vi "config fpga resource.vi"(0 "fifo channel in":refnum<class "fifo channel.lvclass">, 1 "pairs in":T2[](array[typedef]), 2 "tagbus index":i32, 3 "bitfile ref in":refnum<k20>, 4 "hardware resource":T1, 5 "error in (no error)":errorcluster) -> (14 "fifo channel out":refnum<class "fifo channel.lvclass">, 15 "pairs out":T2[](array[typedef]), 19 "error out":errorcluster)   [LabVIEW 2014, in "fifo channel.lvclass"]
uses:
  fifo channel.lvclass
  OLD Project Folder/execution/control index set.ctl
  <vilib>/NI/Tag Bus/tag/Data Type.ctl
  OLD Project Folder/configuration/fpga resource supported data types.ctl
  <vilib>/NI/LVFPGA Adv Session Resources/ResourceInfo.ctl
  <vilib>/NI/Tag Bus/tag/tag descriptor.lvclass/tag descriptor.ctl
  fifo channel.lvclass/fifo channel.ctl
  <vilib>/NI/LVFPGA Adv Session Resources/OpenByNameSubVI.vi
  <vilib>/NI/Tag Bus/tag/read data type.vi
  <vilib>/NI/Tag Bus/tag/read tag name.vi
  Read fifo config.vi
  <vilib>/rvi/interface/common/dynamic/niFpgaEscapeDelimiterAndNull.vi
  <vilib>/Utility/error.llb/Error Cluster From Error Code.vi
  <vilib>/rvi/interface/common/niFpgaWaitOnOcc.vi
  <vilib>/NI/LVFPGA Adv Session Resources/OpenByName.xnode
  <vilib>/rvi/interface/nirviMethod/nirviMethod.xnode
  <vilib>/rvi/errors/niLvFpgaMergeErrorWithErrorCode.vi
  OLD Project Folder/execution/io runtime.lvclass
  fpga channel/fpga channel.lvclass
  <vilib>/NI/Tag Bus/tag/tag descriptor.lvclass
  <vilib>/FPGAPlugInAG/Dynamic/niLvFpga_ConfigureFifo_Dynamic.vi
  <vilib>/FPGAPlugInAG/Dynamic/niLvFpga_StartFifo_Dynamic.vi
  <vilib>/NI/LVFPGA Adv Session Resources/LVFPGAAdvSessionResources.lvlib
  <vilib>/Utility/VariantDataType/VariantType.lvlib
panel:
  out "Actual Depth":u32
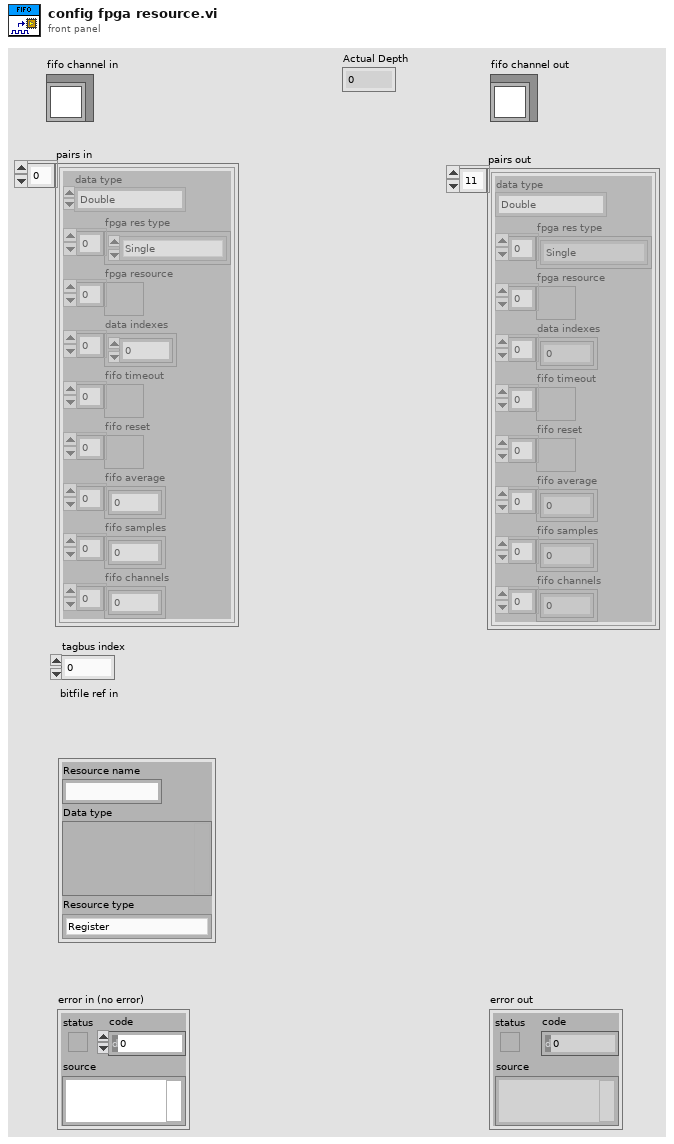
[diagram p1: front panel]
types:
  T1 = typedef "LVFPGAAdvSessionResources.lvlib/ResourceInfo.ctl" = cluster{"Resource name":string, "Data type":variant, "Resource type":enum16{"Register", "Host To Target FIFO", "Target To Host FIFO"}}
  T2 = typedef "io runtime.lvclass/control index set.ctl" = cluster{"data type":T3, "fpga res type":T4[], "fpga resource":refnum<k20>[], "data indexes":i32[], "fifo timeout":refnum<k20>[], "fifo reset":refnum<k20>[], "fifo average":i32[], "fifo samples":u32[], "fifo channels":u32[]}
  T3 = typedef "tag bus.lvlib/tag descriptor.lvclass/Data Type.ctl" = enum16{"Double", "Single", "I64", "I32", "I16", "I8", "U64", "U32", "U16", "U8", "Boolean", "String", "Array of Double", "Array of Single", "Array of I64", "Array of I32", "Array of I16", "Array of I8", "Array of U64", "Array of U32", "Array of U16", "Array of U8", "Array of Boolean", "Array of String"}
  T4 = typedef "fpga channel.lvclass/fpga resource supported data types.ctl" = enum16{"Invalid Type", "Single", "I64", "I32", "I16", "I8", "U64", "U32", "U16", "U8", "Boolean", "FXP I,20,5", "FXP I,24,5", "FXP I,24,10", "Fifo 1023,I16"}
  T5 = typedef "fifo channel.lvclass/fifo channel settings.ctl" = cluster{"Timeout":string, "Reset":string, "Averages":i32, "Samples":u32, "Channels":i32, "Fifo size":u32}
  T6 = cluster{"Name":string, "Depth":u32, "Write? (Deprecated:Use Implementation)":bool, "Physical Channel":u32, "Base Address":u32, "Data Width":u32, "Data Type":enum32{"Boolean", "I8", "I16", "I32", "I64", "U8", "U16", "U32", "U64", "FXP", "CustomControl", "SGL"}, "FXP Properties":variant, "Write Window Address":u32, "Implementation":enum16{"niFpgaTargetToHost", "niFpgaHostToTarget", "niFpgaPeerToPeerWriter", "niFpgaPeerToPeerReader", "niCoreTargetToHost", "niCoreHostToTarget"}, "Control Set":u32}[]
  T7 = cluster{"Name":string, "type":variant, "indicator?":bool}[]
  T8 = typedef "VariantType.lvlib/Type.ctl" = enum8{"Invalid Type", "Void", "I8", "I16", "I32", "I64", "U8", "U16", "U32", "U64", "Single Float", "Double Float", "Extended Float", "Single Complex", "Double Complex", "Extended Complex", "Enum U8", "Enum U16", "Enum U32", "Enum U64", "Single Float With Unit", "Double Float With Unit", "Extended Float With Unit", "Single Complex with Unit", "Double Complex with Unit", "Extended Complex with Unit", "Boolean", "String", "Path", "Picture", "Tag", "Array", "Cluster", "Variant", "LV Variant", "Waveform", "Timestamp", "Digital Waveform", "Digital Data", "ExpressData", "Refnum", "External Data", "VI", "Poly VI", "LabVIEW Class Instance", "Fixed Point"}
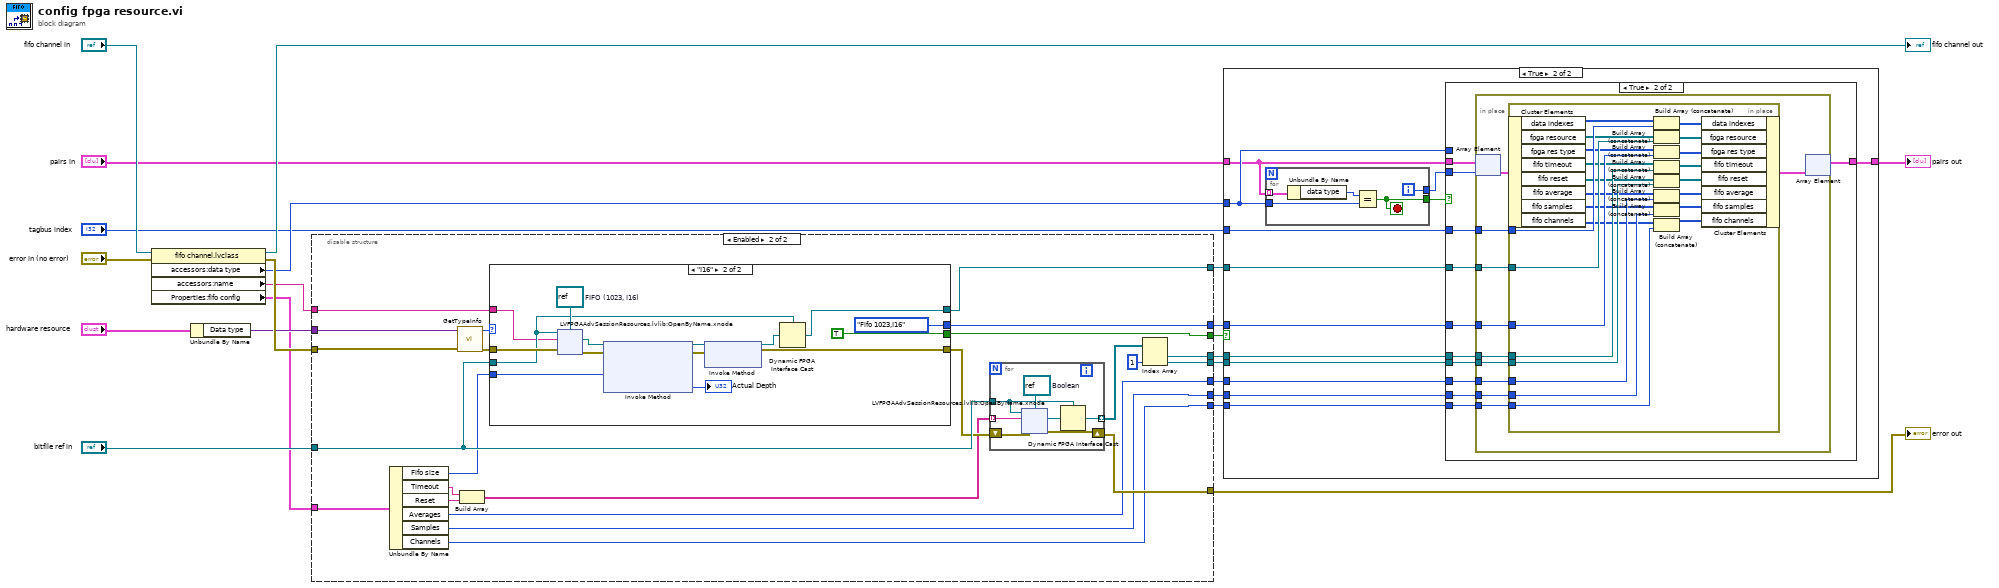
[diagram p0: block diagram]
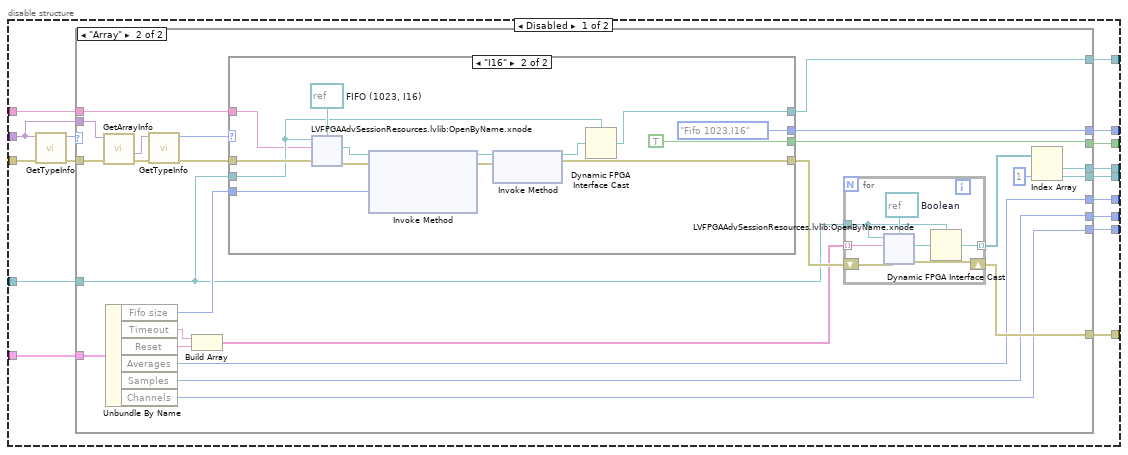
[diagram p2: hidden frame]
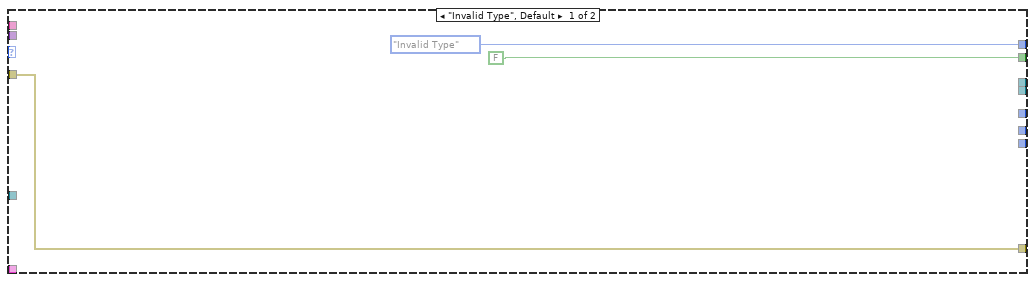
[diagram p3: hidden frame]
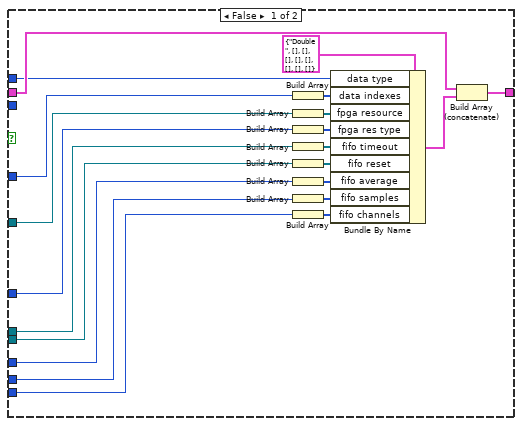
[diagram p7: hidden frame]
diagram:
  n1 = property class="fifo channel.lvclass"(reference="fifo channel in", error in="error in (no error)") -> (reference out=→"fifo channel out":refnum<class "fifo channel.lvclass">, error out=w22:errorcluster, "accessors:data type"=w19:T3, "accessors:name"=w10:string, "Properties:fifo config"=w11:T5)
  n2 = Unbundle By Name("hardware resource") -> ("Data type"=w14:variant)
  n3 = disable-structure shown="Enabled" {
    disable-tunnel: w22 -> [w38 w116]
    disable-tunnel: w14 -> [w36 w117]
    disable-tunnel: "bitfile ref in" -> [w35 w138]
    disable-tunnel: w11 -> [w34 w137]
    disable-tunnel: w10 -> [w33 w136]
    disable-tunnel: [w32 w135] -> w9
    disable-tunnel: [w31 w134] -> w8
    disable-tunnel: [w30 w133] -> w7
    disable-tunnel: [w29 w132] -> w6
    disable-tunnel: [w28 w131] -> w5
    disable-tunnel: [w27 w130] -> w4
    disable-tunnel: [w26 w129] -> w3
    disable-tunnel: [w25 w128] -> w2
    disable-tunnel: [w24 w127] -> w1
    frame Disabled {
      n4 = call <vilib>:"GetTypeInfo.vi"("error in (no error)"=w38, "Variant"=w36) -> ("error out"=w37:errorcluster, "Type Enum"=w23:T8)  [unwired: 5 in, 3 out]
      n5 = case shown="\"Array\"" w23 {
        tunnel: w37 -> [w39 w62]
        tunnel: [FALSE w50] -> w32
        tunnel: w36 -> [_ w61]
        tunnel: w35 -> [_ w53]
        tunnel: [fpga_resource_supported_data_types."Invalid Type" ("fpga res type") w51] -> w29
        tunnel: w34 -> [_ w58]
        tunnel: w33 -> [_ w56]
        tunnel: [_ w52] -> w30
        tunnel: [w39 w49] -> w31
        tunnel: [_ w46] -> w28
        tunnel: [_ w45] -> w27
        tunnel: [_ w44] -> w26
        tunnel: [_ w43] -> w25
        tunnel: [_ w42] -> w24
        frame "Invalid Type", Default {
        }
        frame "Array" {
          n6 = call <vilib>:"GetArrayInfo.vi"("error in (no error)"=w62, "Variant"=w61) -> ("error out"=w64:errorcluster, "ArrayElement"=w63:variant)  [unwired: 6 in, 2 out]
          n7 = Unbundle By Name(w58) -> ("Fifo size"=w57:u32, "Timeout"=w55:string, "Reset"=w54:string, "Averages"=w44:i32, "Samples"=w43:u32, "Channels"=w42:i32)
          n8 = call <vilib>:"GetTypeInfo.vi"("error in (no error)"=w64, "Variant"=w63) -> ("error out"=w60:errorcluster, "Type Enum"=w65:T8)  [unwired: 5 in, 3 out]
          n9 = Build Array(w55, w54) -> (w59:string[])
          n10 = case shown="\"I16\"" w65 {
            tunnel: [_ TRUE] -> w50
            tunnel: w53 -> [_ w93]
            tunnel: w60 -> [w87 w94]
            tunnel: [w87 w92] -> w66
            tunnel: [_ fpga_resource_supported_data_types."Fifo 1023,I16" ("fpga res type")] -> w51
            tunnel: w57 -> [_ w91]
            tunnel: w56 -> [_ w90]
            tunnel: [_ w88] -> w52
            frame "Invalid Type", Default {
            }
            frame "I16" {
              w97 = refnum<k20> refnum  # FIFO (1023, I16)
              n11 = xnode "LVFPGAAdvSessionResources.lvlib:OpenByName.xnode"("FPGA VI Reference in"=w93, "Resource name in"=w90, "Single resource reference type in"=w97, "Error in"=w94) -> ("Single resource reference out"=w95:refnum<k20>, "Error out"=w100:errorcluster)  [unwired: 1 out]
              n12 = xnode "Invoke Method"("FPGA VI Reference In"=w95, "error in"=w100, "Requested Depth"=w91) -> ("FPGA VI Reference Out"=w98:refnum<k20>, "error out"=w99:errorcluster, "Actual Depth"=w89:u32)
              n13 = xnode "Invoke Method"("FPGA VI Reference In"=w98, "error in"=w99) -> ("FPGA VI Reference Out"=w96:refnum<k20>, "error out"=w92:errorcluster)
              n14 = Dynamic FPGA Interface Cast(Session In=w93, Type=w96) -> (Session Out=w88:refnum<k20>)
            }
          }
          n15 = for {
            shift-right: [w70] -> w49
            shift-left: w66 -> [w71]
            tunnel: w59 -> [w69] mode=indexing
            tunnel: [w68] -> w47 mode=indexing
            tunnel: w53 -> [w67]
            w73 = refnum<k20> refnum  # Boolean
            n16 = xnode "LVFPGAAdvSessionResources.lvlib:OpenByName.xnode"("FPGA VI Reference in"=w67, "Resource name in"=w69, "Single resource reference type in"=w73, "Error in"=w71) -> ("Single resource reference out"=w72:refnum<k20>, "Error out"=w70:errorcluster)  [unwired: 1 out]
            n17 = Dynamic FPGA Interface Cast(Session In=w67, Type=w72) -> (Session Out=w68:refnum<k20>)
          }
          n18 = Index Array(array=w47, index #2=1 ("index")) -> (element #1=w46:refnum<k20>, element #2=w45:refnum<k20>)  [unwired: 1 in]
        }
      }
    }
    frame Enabled {
      n19 = Unbundle By Name(w137) -> ("Fifo size"=w122:u32, "Timeout"=w121:string, "Reset"=w120:string, "Averages"=w129:i32, "Samples"=w128:u32, "Channels"=w127:i32)
      n20 = call <vilib>:"GetTypeInfo.vi"("error in (no error)"=w116, "Variant"=w117) -> ("error out"=w124:errorcluster, "Type Enum"=w125:T8)  [unwired: 5 in, 3 out]
      n21 = Build Array(w121, w120) -> (w123:string[])
      n22 = case shown="\"I16\"" w125 {
        tunnel: [_ TRUE] -> w135
        tunnel: w138 -> [_ w165]
        tunnel: w124 -> [w159 w166]
        tunnel: [w159 w164] -> w126
        tunnel: [_ fpga_resource_supported_data_types."Fifo 1023,I16" ("fpga res type")] -> w132
        tunnel: w122 -> [_ w163]
        tunnel: w136 -> [_ w162]
        tunnel: [_ w161] -> w133
        frame "Invalid Type", Default {
        }
        frame "I16" {
          w169 = refnum<k20> refnum  # FIFO (1023, I16)
          n23 = xnode "LVFPGAAdvSessionResources.lvlib:OpenByName.xnode"("FPGA VI Reference in"=w165, "Resource name in"=w162, "Single resource reference type in"=w169, "Error in"=w166) -> ("Single resource reference out"=w167:refnum<k20>, "Error out"=w172:errorcluster)  [unwired: 1 out]
          n24 = xnode "Invoke Method"("FPGA VI Reference In"=w167, "error in"=w172, "Requested Depth"=w163) -> ("FPGA VI Reference Out"=w170:refnum<k20>, "error out"=w171:errorcluster, "Actual Depth"=→"Actual Depth":u32)
          n25 = xnode "Invoke Method"("FPGA VI Reference In"=w170, "error in"=w171) -> ("FPGA VI Reference Out"=w168:refnum<k20>, "error out"=w164:errorcluster)
          n26 = Dynamic FPGA Interface Cast(Session In=w165, Type=w168) -> (Session Out=w161:refnum<k20>)
        }
      }
      n27 = for {
        shift-right: [w142] -> w134
        shift-left: w126 -> [w143]
        tunnel: w123 -> [w141] mode=indexing
        tunnel: [w140] -> w118 mode=indexing
        tunnel: w138 -> [w139]
        w145 = refnum<k20> refnum  # Boolean
        n28 = xnode "LVFPGAAdvSessionResources.lvlib:OpenByName.xnode"("FPGA VI Reference in"=w139, "Resource name in"=w141, "Single resource reference type in"=w145, "Error in"=w143) -> ("Single resource reference out"=w144:refnum<k20>, "Error out"=w142:errorcluster)  [unwired: 1 out]
        n29 = Dynamic FPGA Interface Cast(Session In=w139, Type=w144) -> (Session Out=w140:refnum<k20>)
      }
      n30 = Index Array(array=w118, index #2=1 ("index")) -> (element #1=w131:refnum<k20>, element #2=w130:refnum<k20>)  [unwired: 1 in]
    }
  }
  "error out" <- w8
  n31 = case shown="True" w9 {
    tunnel: [w188 w199] -> w20
    tunnel: w19 -> [_ w198]
    tunnel: "pairs in" -> [w188 w197]
    tunnel: "tagbus index" -> [_ w196]
    tunnel: w7 -> [_ w195]
    tunnel: w6 -> [_ w194]
    tunnel: w5 -> [_ w193]
    tunnel: w4 -> [_ w192]
    tunnel: w3 -> [_ w191]
    tunnel: w2 -> [_ w190]
    tunnel: w1 -> [_ w189]
    frame False {
    }
    frame True {
      n32 = for {
        tunnel: w197 -> [w272] mode=indexing
        tunnel: w198 -> [w270]
        tunnel: [w269] -> w201
        tunnel: [w268] -> w200
        i -> [w269]
        stop <- w268 stop-if-true
        n33 = Unbundle By Name(w272) -> ("data type"=w271:T3)
        n34 = Equal?(x=w271, y=w270) -> (x = y?=w268:bool)
      }
      n35 = case shown="True" w200 {
        tunnel: w197 -> [w222 w233]
        tunnel: [w221 w232] -> w199
        tunnel: w201 -> [_ w231]
        tunnel: w198 -> [w220 _]
        tunnel: w196 -> [w217 w230]
        tunnel: w195 -> [w215 w229]
        tunnel: w194 -> [w213 w228]
        tunnel: w193 -> [w211 w227]
        tunnel: w192 -> [w209 w226]
        tunnel: w191 -> [w207 w225]
        tunnel: w190 -> [w205 w224]
        tunnel: w189 -> [w203 w223]
        frame False {
          n36 = Build Array(w217) -> (w216:i32[])
          n37 = Build Array(w215) -> (w214:refnum<k20>[])
          n38 = Build Array(w213) -> (w212:T4[])
          n39 = Build Array(w211) -> (w210:refnum<k20>[])
          n40 = Build Array(w209) -> (w208:refnum<k20>[])
          n41 = Build Array(w207) -> (w206:i32[])
          n42 = Build Array(w205) -> (w204:u32[])
          n43 = Build Array(w203) -> (w202:i32[])
          n44 = Bundle By Name(cluster=T2 {"data type"=enum."Double", "fpga res type"=[], "fpga resource"=[], "data indexes"=[], "fifo timeout"=[], "fifo reset"=[], "fifo average"=[], "fifo samples"=[], "fifo channels"=[]} ("control index set"), "data type"=w220, "data indexes"=w216, "fpga resource"=w214, "fpga res type"=w212, "fifo timeout"=w210, "fifo reset"=w208, "fifo average"=w206, "fifo samples"=w204, "fifo channels"=w202) -> (w218:T2)
          n45 = Build Array (concatenate)(w222, w218) -> (w221:T2[])
        }
        frame True {
          n46 = in-place {
            in-place-border: w230 -> [w241]
            in-place-border: w229 -> [w240]
            in-place-border: w228 -> [w239]
            in-place-border: w227 -> [w238]
            in-place-border: w226 -> [w237]
            in-place-border: w225 -> [w236]
            in-place-border: w224 -> [w235]
            in-place-border: w223 -> [w234]
            n47 = in-place-array #1(w233, w231) -> (w243:T2)
            n48 = in-place {
              in-place-border: w241 -> [w265]
              in-place-border: w240 -> [w263]
              in-place-border: w239 -> [w260]
              in-place-border: w238 -> [w258]
              in-place-border: w237 -> [w254]
              in-place-border: w236 -> [w251]
              in-place-border: w235 -> [w247]
              in-place-border: w234 -> [w245]
              n49 = in-place-cluster #2(w243) -> ("data indexes"=w267:i32[], "fpga resource"=w264:refnum<k20>[], "fpga res type"=w261:T4[], "fifo timeout"=w257:refnum<k20>[], "fifo reset"=w255:refnum<k20>[], "fifo average"=w252:i32[], "fifo samples"=w249:u32[], "fifo channels"=w246:u32[])
              n50 = Build Array (concatenate)(w267, w265) -> (w266:i32[])
              n51 = Build Array (concatenate)(w264, w263) -> (w262:refnum<k20>[])
              n52 = Build Array (concatenate)(w261, w260) -> (w259:T4[])
              n53 = Build Array (concatenate)(w257, w258) -> (w256:refnum<k20>[])
              n54 = Build Array (concatenate)(w255, w254) -> (w253:refnum<k20>[])
              n55 = Build Array (concatenate)(w252, w251) -> (w250:i32[])
              n56 = Build Array (concatenate)(w249, w247) -> (w248:u32[])
              n57 = Build Array (concatenate)(w246, w245) -> (w244:u32[])
              n58 = in-place-cluster #2("data indexes"=w266, "fpga resource"=w262, "fpga res type"=w259, "fifo timeout"=w256, "fifo reset"=w253, "fifo average"=w250, "fifo samples"=w248, "fifo channels"=w244) -> (w242:T2)
            }
            n59 = in-place-array #1(w242) -> (w232:T2[])  [unwired: 1 out]
          }
        }
      }
    }
  }
  "pairs out" <- w20
